vi "Handle.vi"(8 "error in (no error)":errorcluster, 11 "E55555 in":refnum<class "E55555.lvclass">) -> (0 "error out":errorcluster, 3 "E55555 out":refnum<class "E55555.lvclass">)   [LabVIEW 2022 SP3, in "Demo.lvlib" / "E55555.lvclass"]
uses:
  E55555.lvclass
  C:/Users/jakub/repos/gh/lv-error/Source/Demo/TestApplicationError/TestApplicationError.lvclass
  TestApplicationError/TestApplicationError.lvclass/TestApplicationError.ctl
  TestApplication/TestApplication.lvclass/TestApplication.ctl
  TestApplicationError/Read TestApplication.vi
  TestApplication/Read Events.vi
  TestApplication/TestApplication.lvclass
  E55555.lvclass/E55555.ctl
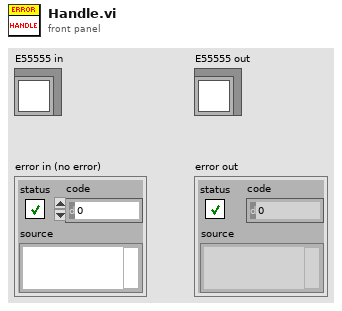
[diagram p1: front panel]
types:
  T1 = typedef "Demo.lvlib/TestApplication.lvclass/_Events.ctl" = cluster{"ToggleLed":refnum<user-event>}
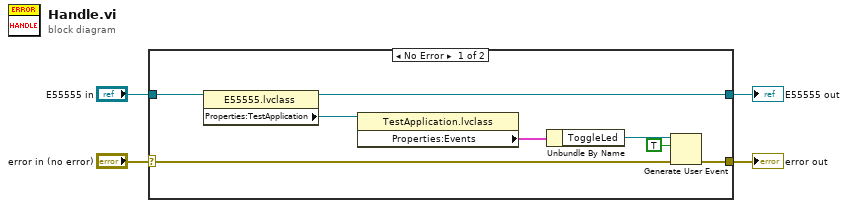
[diagram p0: block diagram]
diagram:
  n1 = case shown="No Error" "error in (no error)" {
    selector: "error in (no error)" -> [w7 w14]
    tunnel: [w6 w14] -> w4
    tunnel: [w11 w13] -> w3
    tunnel: "E55555 in" -> [w12 w13]
    frame No Error {
      n2 = property class="E55555.lvclass"(reference=w12) -> (reference out=w11:refnum<class "E55555.lvclass">, "Properties:TestApplication"=w10:refnum<class "TestApplication.lvclass">)  [unwired: 1 in, 1 out]
      n3 = property class="TestApplication.lvclass"(reference=w10) -> ("Properties:Events"=w9:T1)  [unwired: 1 in, 2 out]
      n4 = Unbundle By Name(w9) -> ("ToggleLed"=w8:refnum<user-event>)
      n5 = Generate User Event(user event=w8, event data cluster=TRUE ("event data"), error in=w7) -> (error out=w6:errorcluster)  [unwired: 1 in, 1 out]
    }
    frame Error {
    }
  }
  "error out" <- w4
  "E55555 out" <- w3
